vi "Read Attributes.vi"(11 "Operation Complete Msg":refnum<class "Operation Complete Msg.lvclass">) -> (2 "Payload":cluster{"Operation Complete":bool})   [LabVIEW 2018, in "Generic Optimization Actor.lvlib" / "Operation Complete Msg.lvclass"]
uses:
  Operation Complete Msg.lvclass
  Operation Complete Msg.lvclass/Operation Complete Msg.ctl
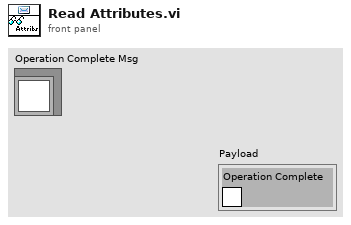
[diagram p1: front panel]
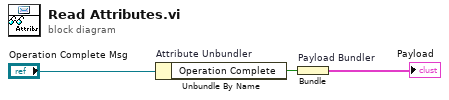
[diagram p0: block diagram]
diagram:
  n1 = Unbundle By Name "Attribute Unbundler"("Operation Complete Msg") -> ("Operation Complete"=w1:bool)
  n2 = Bundle "Payload Bundler"("Operation Complete"=w1) -> (→"Payload":cluster{"Operation Complete":bool})  [unwired: 1 in]
